vi "Launch.vi"(6 "Sequencer":refnum<class "MessageQ.lvclass">, 7 "VolatusAPI":refnum<class "VolatusAPI.lvclass">, 8 "error in (no error)":refnum<class "MultiErrors.lvclass">, 10 "Sequence Config":refnum<class "Sequence Config.lvclass">, 11 "Sequence in":refnum<class "Sequence.lvclass">) -> (0 "error out":refnum<class "MultiErrors.lvclass">, 3 "Sequence out":refnum<class "Sequence.lvclass">)   [LabVIEW 2020, in "VolatusSeq.lvlib" / "Sequence.lvclass"]
uses:
  Sequence.lvclass
  VolatusErrorUtilities/MultiErrors/MultiErrors.lvclass
  Volatus/VolatusAPI/VolatusAPI.lvclass
  VolatusSeqConfig/Sequence Config/Sequence Config.lvclass
  Volatus/MessageQ/MessageQ.lvclass
  lv-promises/Promises/Value/Value.lvclass
  lv-promises/Promises/Promise/Promise.lvclass/Promise.ctl
  lv-promises/Promises/Future/Future.lvclass/Future.ctl
  Loop Async.vi
  lv-promises/Promises/Future/Future.lvclass
  Sequence.lvclass/Sequence.ctl
  lv-promises/Promises/Promise/Promise.lvclass
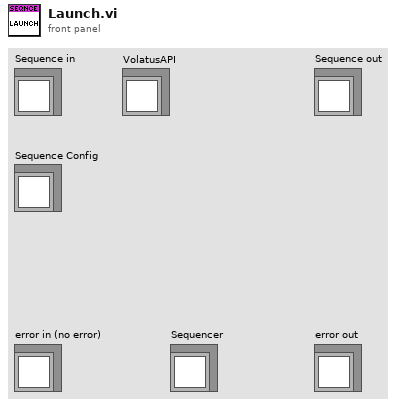
[diagram p1: front panel]
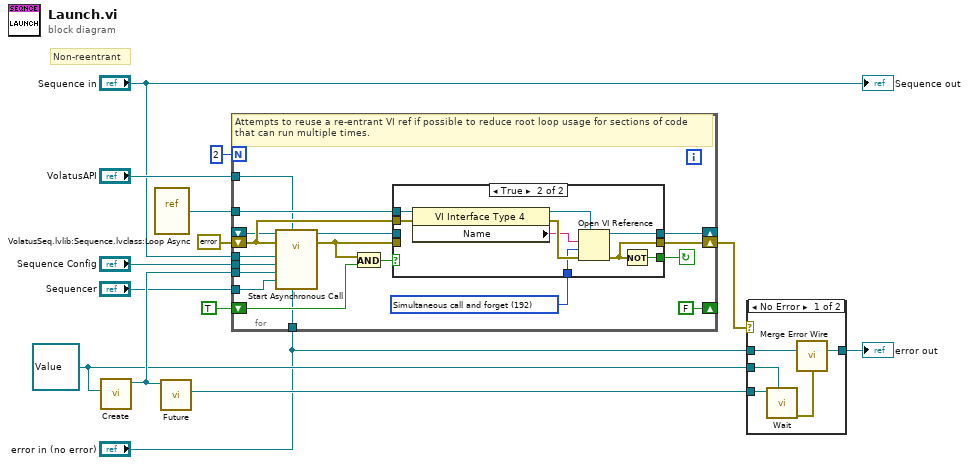
[diagram p0: block diagram]
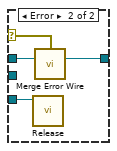
[diagram p3: hidden frame]
diagram:
  w4 = refnum<class "Value.lvclass"> refnum ("Futures:Value.lvclass")
  # "Non-reentrant"
  n1 = call "Create.vi"("Result Type (None)"=w4) -> ("Promise"=w7:refnum<class "Promise.lvclass">)  [unwired: 9 in, 1 out]
  n2 = vi-ref "VolatusSeq.lvlib:Sequence.lvclass:Loop Async.vi"() -> (w12:refnum<vi>)
  n3 = call "Future.vi"("Promise in"=w7) -> ("Future"=w5:refnum<class "Future.lvclass">)  [unwired: 9 in, 1 out]
  n4 = for {
    N: 2 -> [_]
    tunnel: w12 -> [w31]
    shift-right: [w30] -> _
    shift-left: _ -> [w29]
    shift-right: [w27] -> w6
    shift-left: errorcluster {"status"=FALSE, "code"=0, "source"=""} ("error constant") -> [w32]
    shift-right: [FALSE] -> _
    shift-left: TRUE -> [w24]
    tunnel: "VolatusAPI" -> [w21]
    tunnel: "Sequence in" -> [w20]
    tunnel: "Sequence Config" -> [w19]
    tunnel: w7 -> [w18]
    tunnel: "Sequencer" -> [w16]
    tunnel: "error in (no error)" -> [w15]
    stop <- w23 continue-if-true
    w17 = 192 items=["Record modifications"=1, "Open templates for editing"=2, "Prompt user to save"=4, "Prepare for reentrant run"=8, "Prompt to find missing subVIs"=16, "Hide loading dialog box"=32, "Enable simultaneous calls"=64, "Prepare to call and forget"=128, "Simultaneous call and forget"=192, "Prepare to call and collect"=256, "Simultaneous call and collect"=320]
    # "Attempts to reuse a re-entrant VI ref if possible to reduce root loop usage for sections of code that can run multiple times."
    n5 = call-by-ref "Start Asynchronous Call"(reference=w29, error in=w32, "MultiErrors"=w15, "VolatusAPI"=w21, "Sequencer"=w16, "Promise"=w18, "Sequence Config"=w19, "Sequence in"=w20) -> (reference out=w28:refnum<vi>, error out=w26:errorcluster)  [unwired: 6 in]
    n6 = And(x=w26, y=w24) -> (x .and. y?=w25:bool)
    n7 = case shown="True" w25 {
      tunnel: w31 -> [_ w42]
      tunnel: w17 -> [_ w40]
      tunnel: [w34 w38] -> w30
      tunnel: w28 -> [w34 _]
      tunnel: [w33 w36] -> w27
      tunnel: w26 -> [w33 _]
      tunnel: w32 -> [_ w37]
      tunnel: [_ w35] -> w23
      frame False {
      }
      frame True {
        n8 = property class="VI Interface Type 4"(reference=w42, error in=w37) -> (reference out=w39:refnum<vi>, error out=w43:errorcluster, "Name"=w41:string)
        n9 = Open VI Reference(type specifier VI Refnum (for type only)=w39, vi path=w41, options=w40, error in (no error)=w43) -> (vi reference=w38:refnum<vi>, error out=w36:errorcluster)  [unwired: 2 in]
        n10 = Not(x=w36) -> (.not. x?=w35:bool)
      }
    }
  }
  n11 = case shown="No Error" w6 {
    selector: w6 -> [_ w49]
    tunnel: w5 -> [w48 w52]
    tunnel: w4 -> [w47 _]
    tunnel: [w44 w50] -> w1
    tunnel: "error in (no error)" -> [w46 w51]
    frame No Error {
      n12 = call "Wait.vi"("Result Type (None)"=w47, "Future in"=w48) -> ("error out"=w45:errorcluster)  [unwired: 8 in, 1 out]
      n13 = call "Merge Error Wire.vi"("error in (no error)"=w45, "MultiErrors in"=w46) -> ("MultiErrors out"=w44:refnum<class "MultiErrors.lvclass">)  [unwired: 13 in]
    }
    frame Error {
      n14 = call "Release.vi"("Future in"=w52) -> ()  [unwired: 11 in]
      n15 = call "Merge Error Wire.vi"("error in (no error)"=w49, "MultiErrors in"=w51) -> ("MultiErrors out"=w50:refnum<class "MultiErrors.lvclass">)  [unwired: 13 in]
    }
  }
  "error out" <- w1
  "Sequence out" <- "Sequence in"
